vi "Day 2.2 - Calculate postion wth aim.vi"(11 "input":string[](array[string])) -> (3 "output":i32)   [LabVIEW 2021]
uses:
  Controls/submarine position.ctl
panel:
  out "submarine position":T1
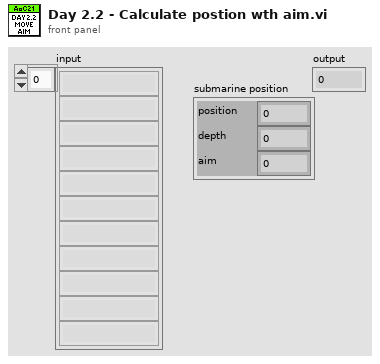
[diagram p1: front panel]
types:
  T1 = typedef "submarine position.ctl" = cluster{"position":i32, "depth":i32, "aim":i32}
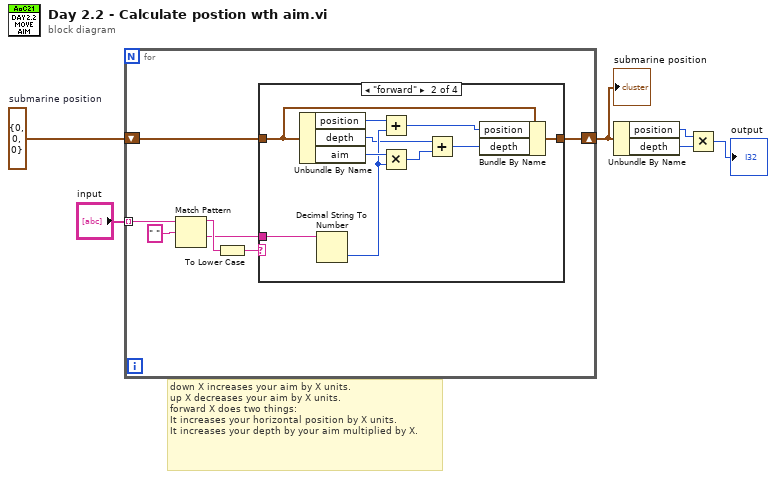
[diagram p0: block diagram]
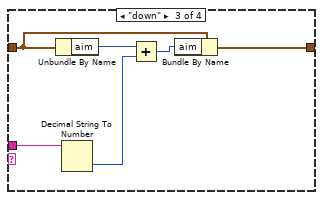
[diagram p3: hidden frame]
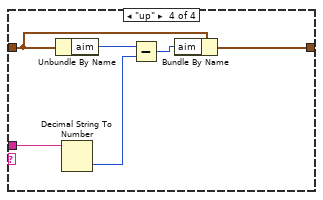
[diagram p4: hidden frame]
diagram:
  w5 = T1 {"position"=0, "depth"=0, "aim"=0}  # submarine position
  # "down X increases your aim by X units.\nup X decreases your aim by X units.\nforward X does two things:\nIt increases your horizontal position by X units.\nIt increases your depth by your aim multiplied by X."
  n1 = for {
    tunnel: "input" -> [w11] mode=indexing
    shift-right: [w12] -> w4
    shift-left: w5 -> [w13]
    n2 = Match Pattern(string=w11, regular expression=" ") -> (before substring=w9:string, after substring=w7:string)  [unwired: 1 in, 2 out]
    n3 = To Lower Case(string=w9) -> (all lower case string=w8:string)
    n4 = case shown="\"forward\"" w8 {
      tunnel: w13 -> [w14 w20 w25 w31]
      tunnel: [w14 w21 w26 w32] -> w12
      tunnel: w7 -> [_ w24 w30 w36]
      frame Default {
      }
      frame "forward" {
        n5 = Unbundle By Name(w20) -> ("position"=w23:i32, "depth"=w17:i32, "aim"=w19:i32)
        n6 = Decimal String To Number(string=w24) -> (number=w18:i32)  [unwired: 2 in, 1 out]
        n7 = Add(x=w23, y=w18) -> (x+y=w22:i32)
        n8 = Multiply(x=w19, y=w18) -> (x*y=w16:i32)
        n9 = Add(x=w17, y=w16) -> (x+y=w15:i32)
        n10 = Bundle By Name(cluster=w20, "position"=w22, "depth"=w15) -> (w21:T1)
      }
      frame "down" {
        n11 = Unbundle By Name(w25) -> ("aim"=w28:i32)
        n12 = Decimal String To Number(string=w30) -> (number=w29:i32)  [unwired: 2 in, 1 out]
        n13 = Add(x=w28, y=w29) -> (x+y=w27:i32)
        n14 = Bundle By Name(cluster=w25, "aim"=w27) -> (w26:T1)
      }
      frame "up" {
        n15 = Unbundle By Name(w31) -> ("aim"=w34:i32)
        n16 = Decimal String To Number(string=w36) -> (number=w35:i32)  [unwired: 2 in, 1 out]
        n17 = Subtract(x=w34, y=w35) -> (x-y=w33:i32)
        n18 = Bundle By Name(cluster=w31, "aim"=w33) -> (w32:T1)
      }
    }
  }
  "submarine position" <- w4
  n19 = Unbundle By Name(w4) -> ("position"=w3:i32, "depth"=w2:i32)
  n20 = Multiply(x=w3, y=w2) -> (x*y=→"output":i32)
